vi "TESTE Main.vi"() -> ()   [LabVIEW 2015]
doc: "Use this template to build a simple state machine design pattern. Each state executes code and determines which state to transition to."
uses:
  controls/TESTE State.ctl
  controls/TESTE Data.ctl
  <vilib>/measure/NI_MABase.lvlib
panel:
  out "Meter":dbl(knob) scale=0.0..10.0
  out "Waveform Graph":dbl[](graph)
  out "Status":string
  in  "phase":dbl format="%.2p"
  in  "amplitude":dbl=1.0 format="%0.2p"
  in  "frequency":dbl=10.0 format="%0.2p"
  in  "signal type":T1(ring)
  in  "Flush Waveform":bool
  in  "Generate Waveform":bool
  in  "Exit":bool
  # "Gerador de Forma de Onda"
  # "Wave Parameters"
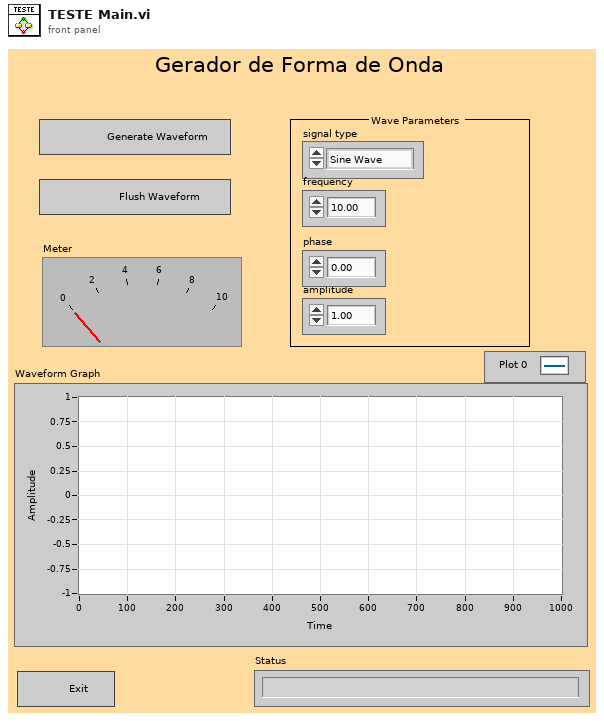
[diagram p1: front panel]
types:
  T1 = enum16{"Sine Wave", "Triangle Wave", "Square Wave", "Sawtooth Wave"}
  T2 = typedef "TESTE Data.ctl" = cluster{"Boolean <Replace Me>":bool, "String <Replace Me>":string, "Data":dbl[]}
  T3 = typedef "TESTE State.ctl" = enum16{"Initialize", "Wait for Event", "Update UI", "Generate Waveform", "Flush Waveform", "Exit"}
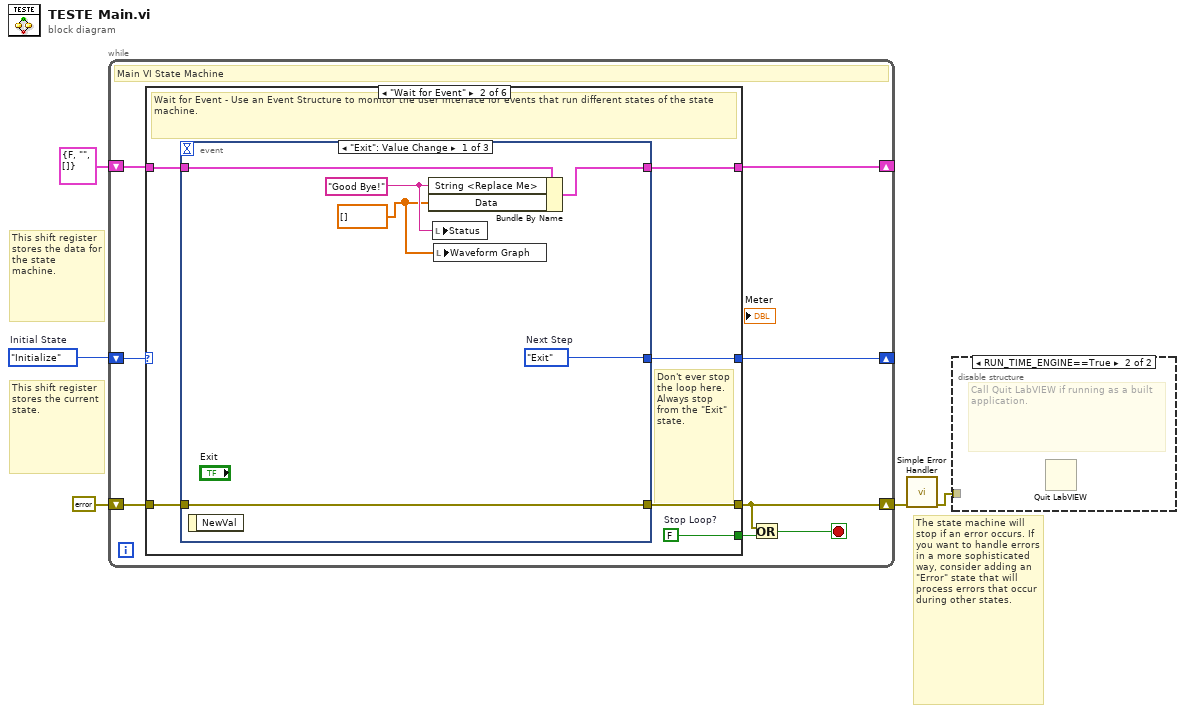
[diagram p0: block diagram]
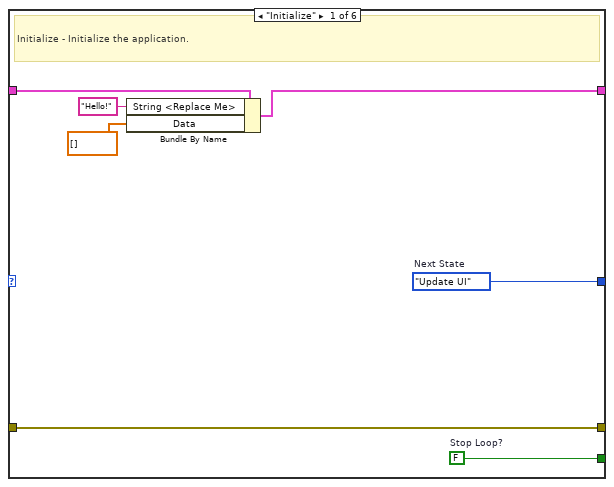
[diagram p3: hidden frame]
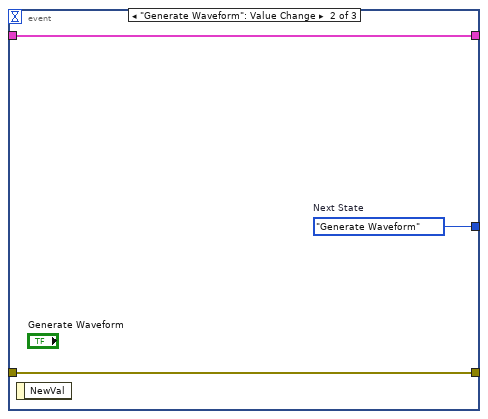
[diagram p4: hidden frame]
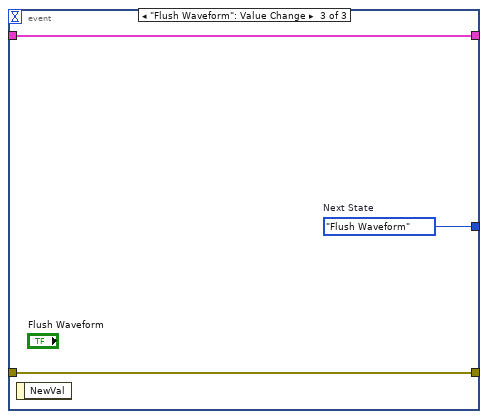
[diagram p5: hidden frame]
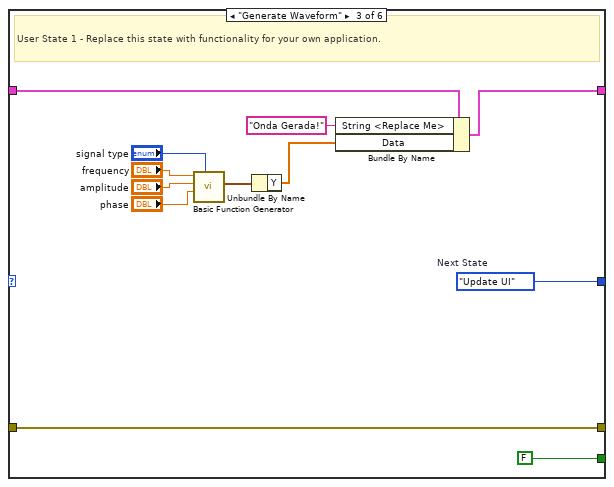
[diagram p6: hidden frame]
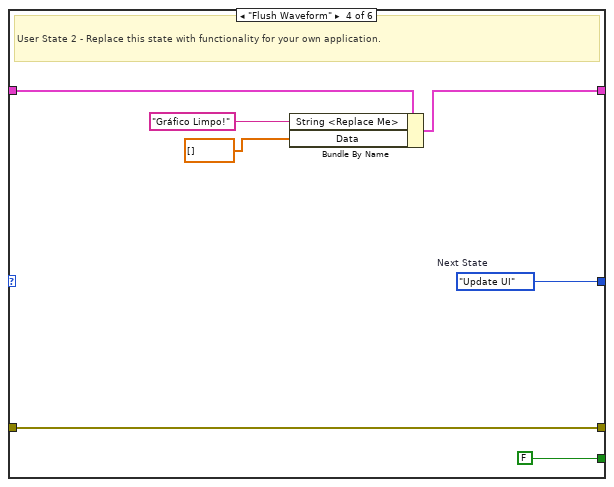
[diagram p7: hidden frame]
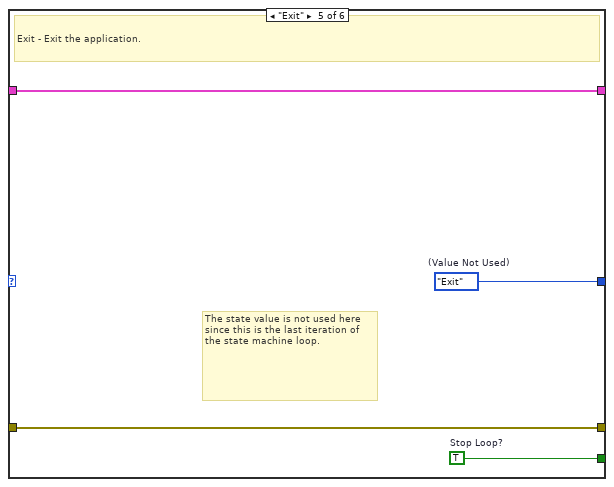
[diagram p8: hidden frame]
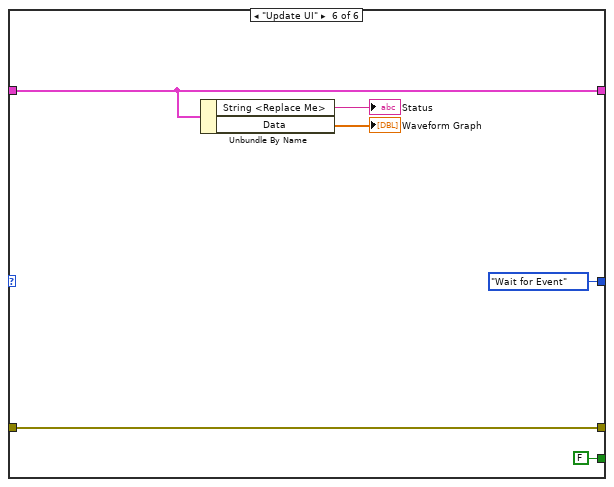
[diagram p9: hidden frame]
diagram:
  w5 = TESTE_State."Initialize"  # Initial State
  # "The state machine will stop if an error occurs. If you want to handle errors in a more sophisticated way, consider adding an \"Error\" state that will process errors that occur during other states."
  # "This shift register stores the data for the state machine."
  # "This shift register stores the current state."
  n1 = while {
    shift-right: [w12] -> _
    shift-left: w5 -> [w13]
    shift-right: [w10] -> _
    shift-left: T2 {"Boolean <Replace Me>"=FALSE, "String <Replace Me>"="", "Data"=[]} ("Data") -> [w11]
    shift-right: [w6] -> w2
    shift-left: errorcluster {"status"=FALSE, "code"=0, "source"=""} ("error constant") -> [w9]
    stop <- w7 stop-if-true
    # "Main VI State Machine"
    n2 = case shown="\"Wait for Event\"" w13 {
      tunnel: [w20 w21 w50 w57 w61 TESTE_State."Wait for Event" ("(Value Not Used)")] -> w12
      tunnel: [w19 w26 FALSE ("Stop Loop?") FALSE ("Stop Loop?") w60 FALSE ("Stop Loop?")] -> w8
      tunnel: w11 -> [w17 w25 w40 w52 w58 w65]
      tunnel: [w16 w22 w39 w51 w58 w65] -> w10
      tunnel: w9 -> [w18 w24 w48 w55 w59 w67]
      tunnel: [w18 w23 w48 w55 w59 w67] -> w6
      frame "Initialize" {
        w19 = FALSE  # Stop Loop?
        w20 = TESTE_State."Update UI"  # Next State
        # "Initialize - Initialize the application."
        n3 = Bundle By Name(cluster=w17, "String <Replace Me>"="Hello!", "Data"=dbl[] []) -> (w16:T2)
      }
      frame "Wait for Event" {
        w26 = FALSE  # Stop Loop?
        # "Don't ever stop the loop here. Always stop from the \"Exit\" state."
        # "Wait for Event - Use an Event Structure to monitor the user interface for events that run different states of the state machine."
        n4 = event shown="[0] \"Exit\": Value Change" {
          selector: _ -> [_ _ _]
          dyn-events: _ -> [_ _ _]
          timeout: _ -> [_ _ _]
          tunnel: [w27 w35 w38] -> w21
          tunnel: w25 -> [w32 w33 w36]
          tunnel: [w30 w33 w36] -> w22
          tunnel: w24 -> [w31 w34 w37]
          tunnel: [w31 w34 w37] -> w23
          event "Exit": Value Change {
            w27 = TESTE_State."Exit"  # Next Step
            w28 = dbl[] [] ("Data")
            w29 = "Good Bye!" ("String <Replace Me>")
            n5 = event-data() -> ()  [unwired: 1 in, 1 out]
            n6 = Bundle By Name(cluster=w32, "String <Replace Me>"=w29, "Data"=w28) -> (w30:T2)
            n7 = local write "Status"(w29) -> ()
            n8 = local write "Waveform Graph"(w28) -> ()
          }
          event "Generate Waveform": Value Change {
            w35 = TESTE_State."Generate Waveform"  # Next State
            n9 = event-data() -> ()  [unwired: 1 in, 1 out]
          }
          event "Flush Waveform": Value Change {
            w38 = TESTE_State."Flush Waveform"  # Next State
            n10 = event-data() -> ()  [unwired: 1 in, 1 out]
          }
        }
      }
      frame "Generate Waveform" {
        w50 = TESTE_State."Update UI"  # Next State
        # "User State 1 - Replace this state with functionality for your own application."
        n11 = call <vilib>:"Basic Function Generator.vi"("signal type"="signal type", "phase"="phase", "amplitude"="amplitude", "frequency"="frequency") -> ("signal out"=w47:waveform(dbl))  [unwired: 5 in, 2 out]
        n12 = Unbundle By Name(w47) -> ("Y"=w46:dbl[])
        n13 = Bundle By Name(cluster=w40, "String <Replace Me>"="Onda Gerada!", "Data"=w46) -> (w39:T2)
      }
      frame "Flush Waveform" {
        w57 = TESTE_State."Update UI"  # Next State
        # "User State 2 - Replace this state with functionality for your own application."
        n14 = Bundle By Name(cluster=w52, "String <Replace Me>"="Gráfico Limpo!" ("Running User State 2"), "Data"=dbl[] []) -> (w51:T2)
      }
      frame "Exit" {
        w60 = TRUE  # Stop Loop?
        w61 = TESTE_State."Exit"  # (Value Not Used)
        # "The state value is not used here since this is the last iteration of the state machine loop."
        # "Exit - Exit the application."
      }
      frame "Update UI" {
        n15 = Unbundle By Name(w65) -> ("String <Replace Me>"=→"Status":string, "Data"=→"Waveform Graph":dbl[])
      }
    }
    n16 = Or(x=w6, y=w8) -> (x .or. y?=w7:bool)
  }
  n17 = call <vilib>:"Simple Error Handler.vi"("error in (no error)"=w2) -> ("error out"=w1:errorcluster)  [unwired: 4 in, 4 out]
  n18 = disable-structure shown="RUN_TIME_ENGINE==True" {
    disable-tunnel: w1 -> [_ _]
    frame condition #0 (active) {
    }
    frame condition #1 {
      # "Call Quit LabVIEW if running as a built application."
      n19 = Quit LabVIEW() -> ()  [unwired: 1 in]
    }
  }
